vi "Test shm get Event log Level LV.vi"(8 "error in (no error)":errorcluster, 11 "logevent_logLevel_Ctl":cluster{"level":i32, "priority":i32}) -> (0 "error out":errorcluster, 2 "function return":i32, 3 "logevent_logLevel_Ctl out":cluster{"level":i32, "priority":i32})   [LabVIEW 2018, in "SALLV_Test.lvlib"]
doc: "int Test_shm_getEvent_logLevelLV(Test_logevent_logLevelLV *logevent_logLevel_Ctl );"
uses:
  SALLV_Test.lvlib
  SALLV_Test.so
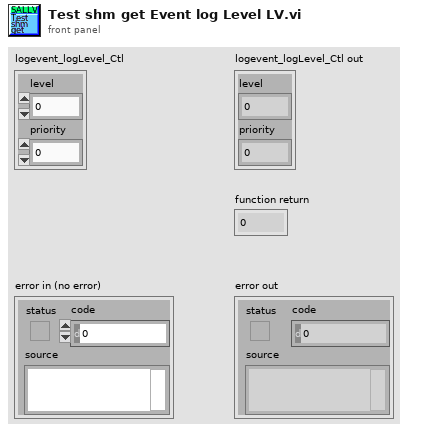
[diagram p1: front panel]
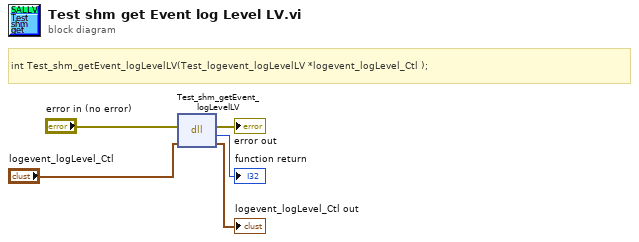
[diagram p0: block diagram]
diagram:
  # "int Test_shm_getEvent_logLevelLV(Test_logevent_logLevelLV *logevent_logLevel_Ctl );"
  n1 = dll-call lib="home/ttsai/Documents/salLabVIEWtestData/SALLV_Test.*" fn="Test_shm_getEvent_logLevelLV"(error in="error in (no error)", "logevent_logLevel_Ctl"="logevent_logLevel_Ctl") -> (error out=→"error out":errorcluster, →"function return":i32, "logevent_logLevel_Ctl"=→"logevent_logLevel_Ctl out":cluster{"level":i32, "priority":i32})  [unwired: 2 in, 1 out]
